vi "add_message.vi"(8 "error in (no error)":errorcluster, 9 "message_text.lvclass":refnum<class "message_text.lvclass">, 10 "Chat Session Name":string="default", 11 "simple_html_chat_ui in":refnum<class "simple_html_chat_ui.lvclass">) -> (0 "error out":errorcluster, 3 "simple_html_chat_ui out":refnum<class "simple_html_chat_ui.lvclass">)   [LabVIEW 2020, in "simple_html_chat_ui.lvclass"]
uses:
  simple_html_chat_ui.lvclass
  src/models/message_text/message_text.lvclass
  simple_html_chat_ui.lvclass/simple_html_chat_ui.ctl
  <vilib>/httpClient/POSTBuffer.vi
  <vilib>/httpClient/LabVIEWHTTPClient.lvlib
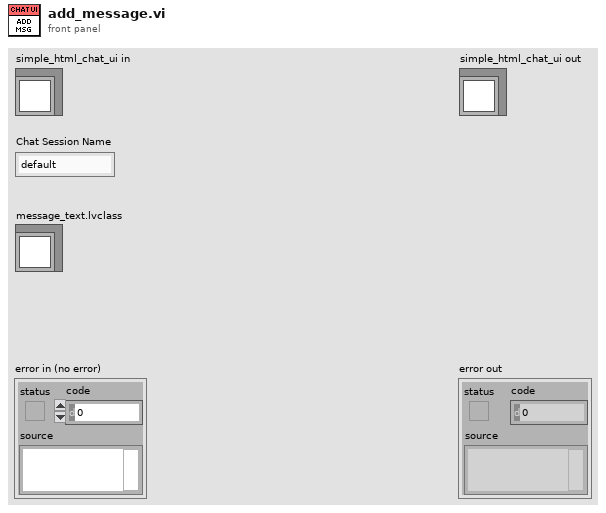
[diagram p1: front panel]
types:
  T1 = cluster{"session":string, "role":string, "message":string}
  T2 = typedef "message_text.lvclass/message.ctl" = cluster{"role":string, "content":string[]}
  T3 = typedef "LabVIEWHTTPClient.lvlib/ClientHandle.ctl" = refnum<k1>
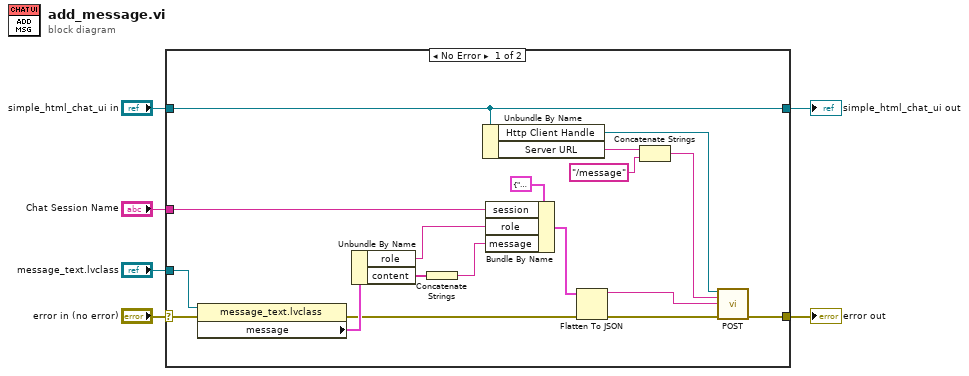
[diagram p0: block diagram]
diagram:
  n1 = case shown="No Error" "error in (no error)" {
    selector: "error in (no error)" -> [w22 w26]
    tunnel: [w10 w26] -> w5
    tunnel: [w14 w25] -> w3
    tunnel: "simple_html_chat_ui in" -> [w14 w25]
    tunnel: "Chat Session Name" -> [w23 _]
    tunnel: "message_text.lvclass" -> [w21 _]
    frame No Error {
      n2 = property class="message_text.lvclass"(reference=w21, error in=w22) -> (error out=w16:errorcluster, "message"=w20:T2)  [unwired: 1 out]
      n3 = Unbundle By Name(w20) -> ("role"=w19:string, "content"=w18:string[])
      n4 = Concatenate Strings(w18) -> (w17:string)
      n5 = Unbundle By Name(w14) -> ("Http Client Handle"=w9:T3, "Server URL"=w13:string)
      n6 = Bundle By Name(cluster=T1 {"session"="", "role"="", "message"=""}, "session"=w23, "role"=w19, "message"=w17) -> (w15:T1)
      n7 = Flatten To JSON(anything=w15, error in (no error)=w16) -> (JSON string=w7:string, 11:w11:errorcluster)  [unwired: 1 in]
      n8 = Concatenate Strings(w13, "/message" ("string")) -> (w8:string)
      n9 = call-poly <vilib>:"POST.vi"("client handle"=w9, "url"=w8, "buffer"=w7, "error in (no error)"=w11) -> ("error out"=w10:errorcluster)  [unwired: 8 in, 3 out]
    }
    frame Error {
    }
  }
  "error out" <- w5
  "simple_html_chat_ui out" <- w3
